vi "Test.vi"() -> ()   [LabVIEW 2016]
doc: "This VI is called when test mode begins, and will automatically be terminated when it ends. You can add manual or automatic tests and invoke them from the dashboard."
uses:
  Globals/InputValues.vi
panel:
  out "Position servo":dbl=0.5
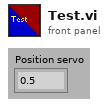
[diagram p1: front panel]
types:
  T1 = typedef "WPI_ServoDeviceRef.ctl" = cluster{"DeviceStatus":errorcluster, "PWM Channel":T2, "DeadBand":T3}
  T2 = typedef "FPGA_DIOPWMChannel.ctl" = enum8{"PWM 0", "PWM 1", "PWM 2", "PWM 3", "PWM 4", "PWM 5", "PWM 6", "PWM 7", "PWM 8", "PWM 9", "PWM MXP 0", "PWM MXP 1", "PWM MXP 2", "PWM MXP 3", "PWM MXP 4", "PWM MXP 5", "PWM MXP 6", "PWM MXP 7", "PWM MXP 8", "PWM MXP 9", "Invalid"}
  T3 = typedef "WPI_PWMDeadband.ctl" = cluster{"Name":string, "maxPositivePwm":i32, "minPositivePwm":i32, "centerPwm":i32, "maxNegativePwm":i32, "minNegativePwm":i32, "angularRange":u16}
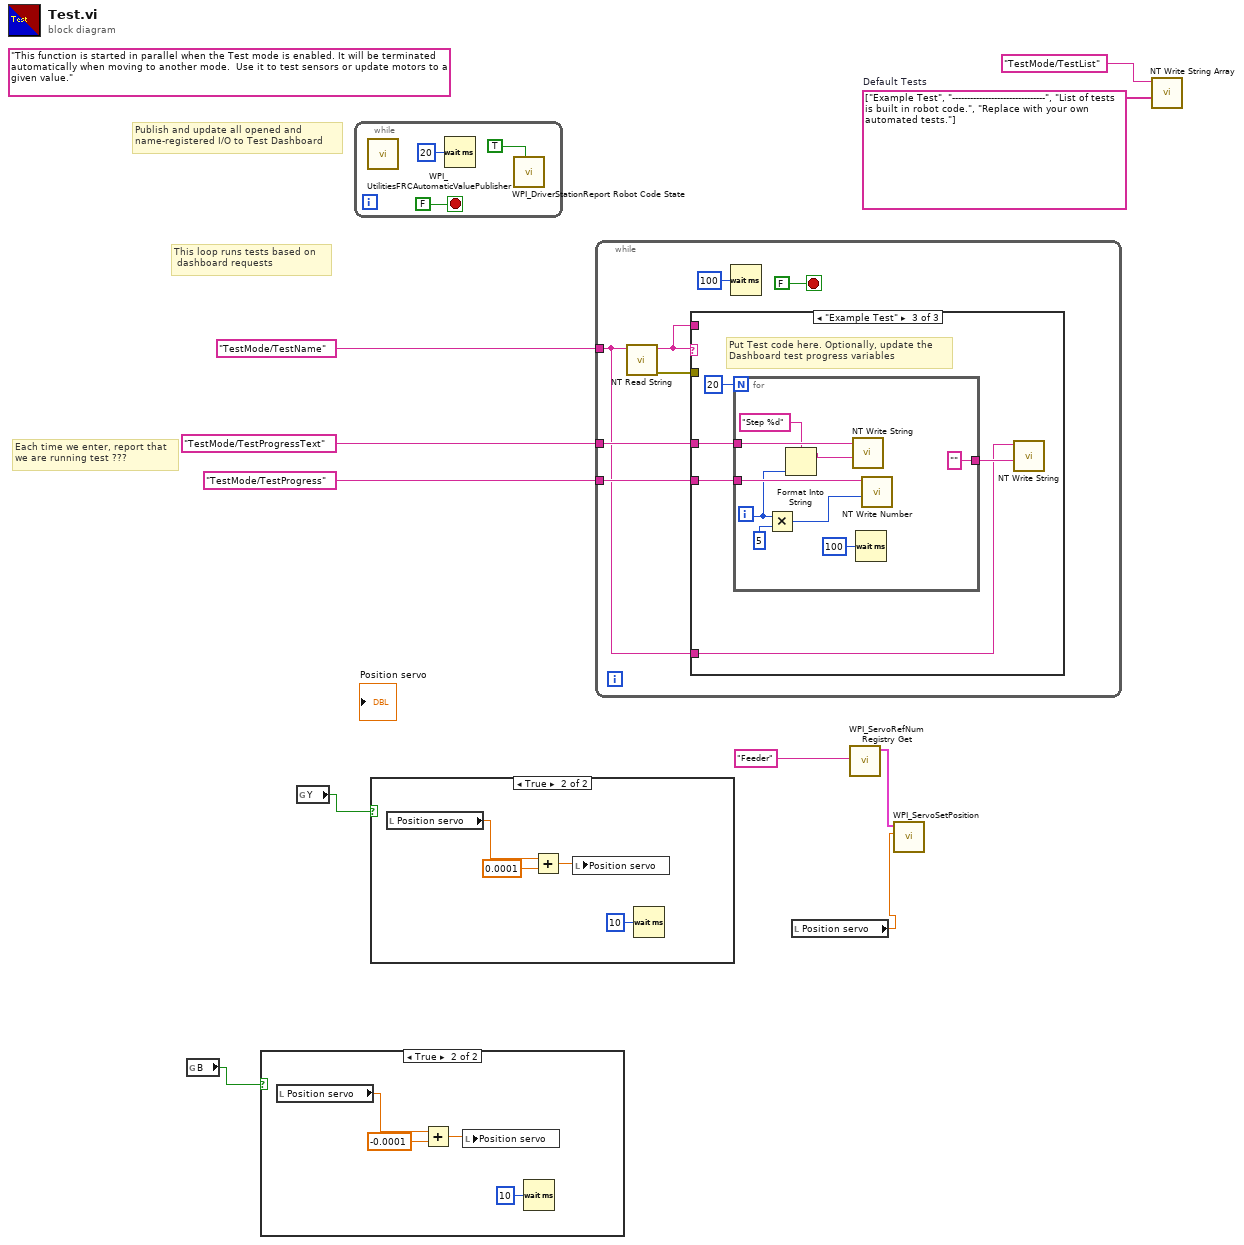
[diagram p0: block diagram]
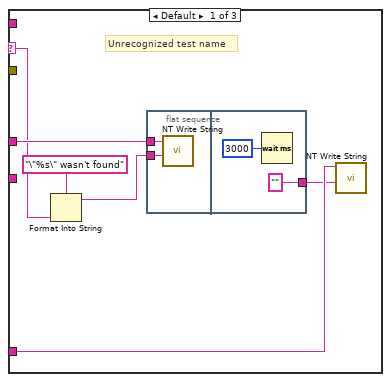
[diagram p4: hidden frame]
diagram:
  w7 = string[] ["Example Test", "-------------------------------", "List of tests is built in robot code.", "Replace with your own automated tests."]  # Default Tests
  (unwired) "This function is started in parallel when the Test mode is enabled. It will be terminated automatically when moving to another mode.  Use it to test sensors or update motors to a given value."
  # "This loop runs tests based on \n dashboard requests"
  # "Publish and update all opened and\nname-registered I/O to Test Dashboard"
  # "Each time we enter, report that\nwe are running test ???"
  n1 = global read "InputValues.vi" "B"() -> (w1:bool)
  n2 = case shown="True" w1 {
    frame False {
    }
    frame True {
      n3 = local read "Position servo"() -> (w14:dbl)
      n4 = Add(x=w14, y=-0.0001) -> (x+y=w11:dbl)
      n5 = local write "Position servo"(w11) -> ()
      n6 = Wait (ms)(milliseconds to wait=u32 10) -> ()  [unwired: 1 out]
    }
  }
  n7 = global read "InputValues.vi" "Y"() -> (w5:bool)
  n8 = while {
    stop <- FALSE stop-if-true
    n9 = call <vilib>:"WPI_UtilitiesFRCAutomaticValuePublisher.vi"() -> ()  [unwired: 12 in]
    n10 = Wait (ms)(milliseconds to wait=u32 20) -> ()  [unwired: 1 out]
    n11 = call <vilib>:"WPI_DriverStationReport Robot Code State.vi"("Test"=TRUE ("Autonomous")) -> ()  [unwired: 10 in, 1 out]
  }
  n12 = case shown="True" w5 {
    frame False {
    }
    frame True {
      n13 = local read "Position servo"() -> (w21:dbl)
      n14 = Add(x=w21, y=0.0001) -> (x+y=w18:dbl)
      n15 = local write "Position servo"(w18) -> ()
      n16 = Wait (ms)(milliseconds to wait=u32 10) -> ()  [unwired: 1 out]
    }
  }
  n17 = while {
    tunnel: "TestMode/TestName" ("Name") -> [w23]
    tunnel: "TestMode/TestProgressText" ("Name") -> [w26]
    tunnel: "TestMode/TestProgress" ("Name") -> [w25]
    stop <- FALSE stop-if-true
    n18 = call <vilib>:"NT Read String.vi"("Name"=w23) -> ("error out"=w22:errorcluster, "String"=w24:string)  [unwired: 9 in]
    n19 = case shown="\"Example Test\"" w24 {
      selector: w24 -> [w33 _ _]
      tunnel: w23 -> [w30 _ w39]
      tunnel: w26 -> [w34 _ w42]
      tunnel: w25 -> [_ _ w43]
      tunnel: w24 -> [_ _ _]
      tunnel: w22 -> [_ _ _]
      frame Default {
        # "Unrecognized test name"
        n20 = Format Into String(format string="\"%s\" wasn't found" ("Name"), w33) -> (resulting string=w32:string)  [unwired: 2 in, 1 out]
        n21 = flat-sequence {
          tunnel: w34 -> [w35]
          tunnel: w32 -> [w36]
          tunnel: ["" ("Name")] -> w29
          frame #0 {
            n22 = call <vilib>:"NT Write String.vi"("String"=w36, "Name"=w35) -> ()  [unwired: 9 in, 1 out]
          }
          frame #1 {
            n23 = Wait (ms)(milliseconds to wait=u32 3000) -> ()  [unwired: 1 out]
          }
        }
        n24 = call <vilib>:"NT Write String.vi"("String"=w29, "Name"=w30) -> ()  [unwired: 9 in, 1 out]
      }
      frame "" {
        # "No test to run"
      }
      frame "Example Test" {
        # "Put Test code here. Optionally, update the\nDashboard test progress variables"
        n25 = for {
          N: 20 -> [_]
          tunnel: w43 -> [w52]
          tunnel: w42 -> [w50]
          tunnel: ["" ("String")] -> w40
          i -> [w47]
          n26 = Multiply(x=w47, y=u32 5 ("milliseconds to wait")) -> (x*y=w48:u32)
          n27 = Format Into String(format string="Step %d", w47) -> (resulting string=w45:string)  [unwired: 2 in, 1 out]
          n28 = call <vilib>:"NT Write String.vi"("String"=w45, "Name"=w50) -> ()  [unwired: 9 in, 1 out]
          n29 = Wait (ms)(milliseconds to wait=u32 100) -> ()  [unwired: 1 out]
          n30 = call <vilib>:"NT Write Number.vi"("Numeric"=w48, "Name"=w52) -> ()  [unwired: 9 in, 1 out]
        }
        n31 = call <vilib>:"NT Write String.vi"("String"=w40, "Name"=w39) -> ()  [unwired: 9 in, 1 out]
      }
    }
    n32 = Wait (ms)(milliseconds to wait=u32 100) -> ()  [unwired: 1 out]
  }
  n33 = local read "Position servo"() -> (w2:dbl)
  n34 = call <vilib>:"WPI_ServoRefNum Registry Get.vi"("refnum name"="Feeder") -> ("ServoDeviceRef"=w3:T1)  [unwired: 9 in, 1 out]
  n35 = call <vilib>:"WPI_ServoSetPosition.vi"("Position"=w2, "ServoDeviceRef"=w3) -> ()  [unwired: 8 in, 2 out]
  n36 = call <vilib>:"NT Write String Array.vi"("String Array"=w7, "Name"="TestMode/TestList") -> ()  [unwired: 9 in, 1 out]
